vi "EnqueueDependencyByPath.vi"(8 "error in (no error)":errorcluster, 9 "Shallow deps?":bool, 10 "Path":path, 11 "CDependencyQueue in":refnum<class "CDependencyQueue.lvclass">) -> (0 "error out":errorcluster, 3 "CDependencyQueue out":refnum<class "CDependencyQueue.lvclass">)   [LabVIEW 2020, in "DependencyInspection.lvlib" / "CDependencyQueue.lvclass"]
uses:
  CDependencyQueue.lvclass
  CDependencyQueue.lvclass/CDependencyQueue.ctl
  DependencyQueue.ctl
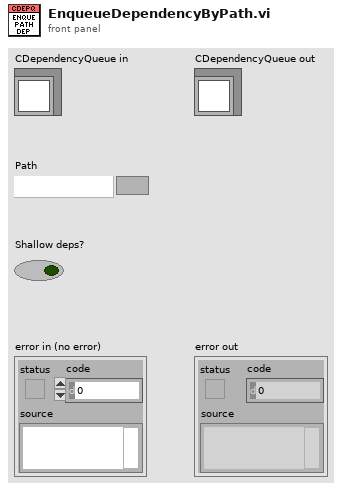
[diagram p1: front panel]
types:
  T1 = typedef "DependencyInspection.lvlib/CDependencyQueue.lvclass/DependencyQueue.ctl" = cluster{"New dependency":path, "Shallow dep?":bool}
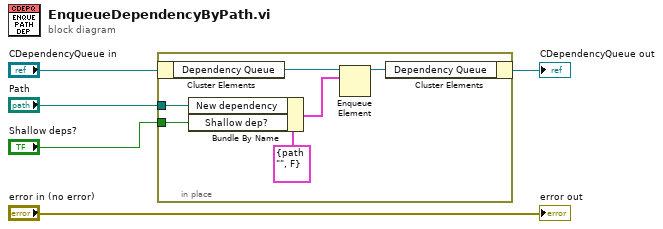
[diagram p0: block diagram]
diagram:
  n1 = in-place {
    in-place-border: "Path" -> [w8]
    in-place-border: "Shallow deps?" -> [w7]
    n2 = in-place-cluster #1("CDependencyQueue in") -> ("Dependency Queue"=w11:refnum<queue>)
    n3 = Bundle By Name(cluster=T1 {"New dependency"=path "", "Shallow dep?"=FALSE} ("Dep info"), "New dependency"=w8, "Shallow dep?"=w7) -> (w6:T1)
    n4 = Enqueue Element(queue=w11, element=w6) -> (queue out=w10:refnum<queue>)  [unwired: 2 in, 2 out]
    n5 = in-place-cluster #1("Dependency Queue"=w10) -> (→"CDependencyQueue out":refnum<class "CDependencyQueue.lvclass">)
  }
  "error out" <- "error in (no error)"
